vi "Contex Menu Selection.vi"(8 "error in (no error)":errorcluster, 10 "MenuItem":string, 11 "HIJ IMAQdx Display in":refnum<class "HIJ IMAQdx Display.lvclass">) -> (0 "error out":errorcluster, 3 "HIJ IMAQdx Display out":refnum<class "HIJ IMAQdx Display.lvclass">)   [LabVIEW 2020, in "HIJ IMAQdx Display.lvlib" / "HIJ IMAQdx Display.lvclass"]
uses:
  HIJ IMAQdx Display.lvclass
  C:/Program Files (x86)/National Instruments/LabVIEW 2020/vi.lib/ActorFramework/Actor/Actor.lvclass
  <vilib>/ActorFramework/Actor/Actor.lvclass/Actor.ctl
  <vilib>/ActorFramework/Message Enqueuer/Message Enqueuer.lvclass/Message Enqueuer.ctl
  <vilib>/ActorFramework/Message Enqueuer/Enqueue.vi
  Application Base Actors/HIJ Vision Camera App/HIJ Vision Camera App Messages/Set BG Image Msg/Set BG Image Msg.lvclass
  C:/Program Files (x86)/National Instruments/LabVIEW 2020/vi.lib/ActorFramework/Message/Message.lvclass
  Application Base Actors/HIJ Vision Application/HIJ Vision Application Messages/Save Image Msg/Save Image Msg.lvclass
  <vilib>/ActorFramework/Message Priority Queue/Priority Enqueue.vi
  HIJ Vision Display/HIJ Vision Display/HIJ Vision Display.lvclass
  <vilib>/ActorFramework/Actor/Actor.lvclass
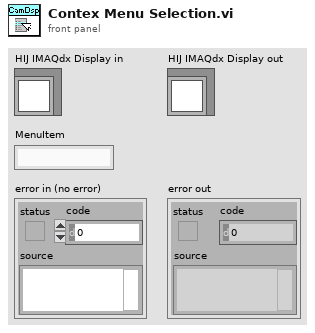
[diagram p1: front panel]
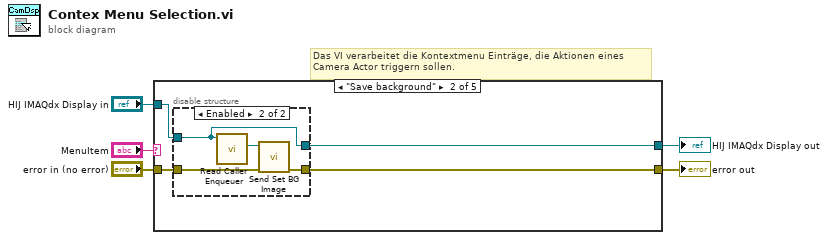
[diagram p0: block diagram]
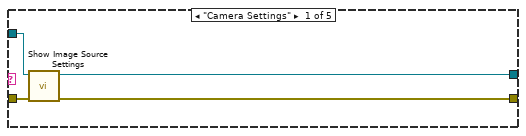
[diagram p2: hidden frame]
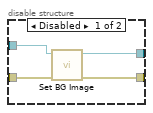
[diagram p3: hidden frame]
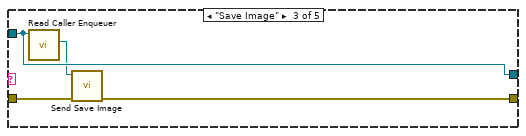
[diagram p4: hidden frame]
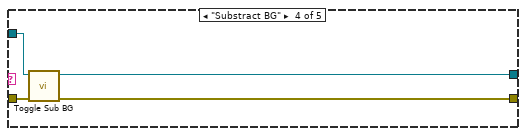
[diagram p5: hidden frame]
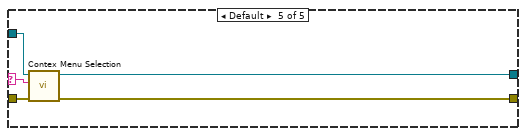
[diagram p6: hidden frame]
diagram:
  # "Das VI verarbeitet die Kontextmenu Einträge, die Aktionen eines \nCamera Actor triggern sollen."
  n1 = case shown="\"Save background\"" "MenuItem" {
    selector: "MenuItem" -> [_ _ _ _ w31]
    tunnel: "HIJ IMAQdx Display in" -> [w9 w13 w25 w29 w34]
    tunnel: "error in (no error)" -> [w8 w11 w22 w26 w33]
    tunnel: [w6 w12 w25 w28 w32] -> w3
    tunnel: [w7 w10 w23 w27 w30] -> w1
    frame "Camera Settings" {
      n2 = call-dynamic "Show Image Source Settings.vi"("error in (no error)"=w8, "AF IMAQ Display in"=w9) -> ("error out"=w7:errorcluster, "AF IMAQ Display out"=w6:refnum<class "HIJ IMAQdx Display.lvclass">)  [unwired: 8 in]
    }
    frame "Save background" {
      n3 = disable-structure shown="Enabled" {
        disable-tunnel: w13 -> [w17 w21]
        disable-tunnel: [w16 w21] -> w12
        disable-tunnel: w11 -> [w15 w19]
        disable-tunnel: [w14 w18] -> w10
        frame Disabled {
          n4 = call "Set BG Image.vi"("error in (no error)"=w15, "IMAQ Display in"=w17) -> ("error out"=w14:errorcluster, "IMAQ Display out"=w16:refnum<class "HIJ IMAQdx Display.lvclass">)  [unwired: 8 in]
        }
        frame Enabled {
          n5 = call <vilib>:"Read Caller Enqueuer.vi"("Actor"=w21) -> ("Caller Enqueuer"=w20:refnum<class "Message Enqueuer.lvclass">)  [unwired: 10 in]
          n6 = call "Send Set BG Image.vi"("error in (no error)"=w19, "Message Enqueuer"=w20) -> ("error out"=w18:errorcluster)  [unwired: 8 in, 1 out]
        }
      }
    }
    frame "Save Image" {
      n7 = call <vilib>:"Read Caller Enqueuer.vi"("Actor"=w25) -> ("Caller Enqueuer"=w24:refnum<class "Message Enqueuer.lvclass">)  [unwired: 10 in]
      n8 = call "Send Save Image.vi"("error in (no error)"=w22, "Message Enqueuer"=w24) -> ("error out"=w23:errorcluster)  [unwired: 8 in, 1 out]
    }
    frame "Substract BG" {
      n9 = call "Toggle Sub BG.vi"("error in (no error)"=w26, "IMAQ Display in"=w29) -> ("error out"=w27:errorcluster, "IMAQ Display out"=w28:refnum<class "HIJ IMAQdx Display.lvclass">)  [unwired: 8 in]
    }
    frame Default {
      n10 = call-parent "Contex Menu Selection.vi"("error in (no error)"=w33, "MenuItem"=w31, "HIJ Vision Display in"=w34) -> ("error out"=w30:errorcluster, "HIJ Vision Display out"=w32:refnum<class "HIJ IMAQdx Display.lvclass">)  [unwired: 7 in]
    }
  }
  "error out" <- w1
  "HIJ IMAQdx Display out" <- w3
